vi "COD质控流程 (子VI).vi"(9 "CODMn量程切换":enum32{"H", "L", "AUTO"}(ring)=enum."AUTO", 10 "CODMn":bool) -> (3 "布尔":bool)   [LabVIEW 2016, in "质控单元.lvlib"]
panel:
  out "CODMn中断报警":bool
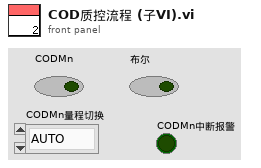
[diagram p1: front panel]
types:
  T1 = enum16{"待机", "启动水样测量", "水样测量中", "启动加标", "启动加标回收", "加标回收测量中", "结束"}
  T2 = cluster{"测量模式":enum16{"水样测量", "标样核查", "零点核查", "跨度核查", "空白测试", "加标回收", "平行样", "校零", "校标"}}
  T3 = enum16{"空闲", "水样测试", "标样核查", "零点核查", "跨度核查", "空白测试", "平行样测试", "质控样", "空白校准", "标样校准", "加标回收"}
  T4 = cluster{"量程":dbl, "检出限":dbl, "加标前水样浓度":dbl, "加标后水样浓度":dbl, "加标水杯定容体积":dbl, "加标母液浓度":dbl, "加标体积":dbl, "加标回收率":dbl}
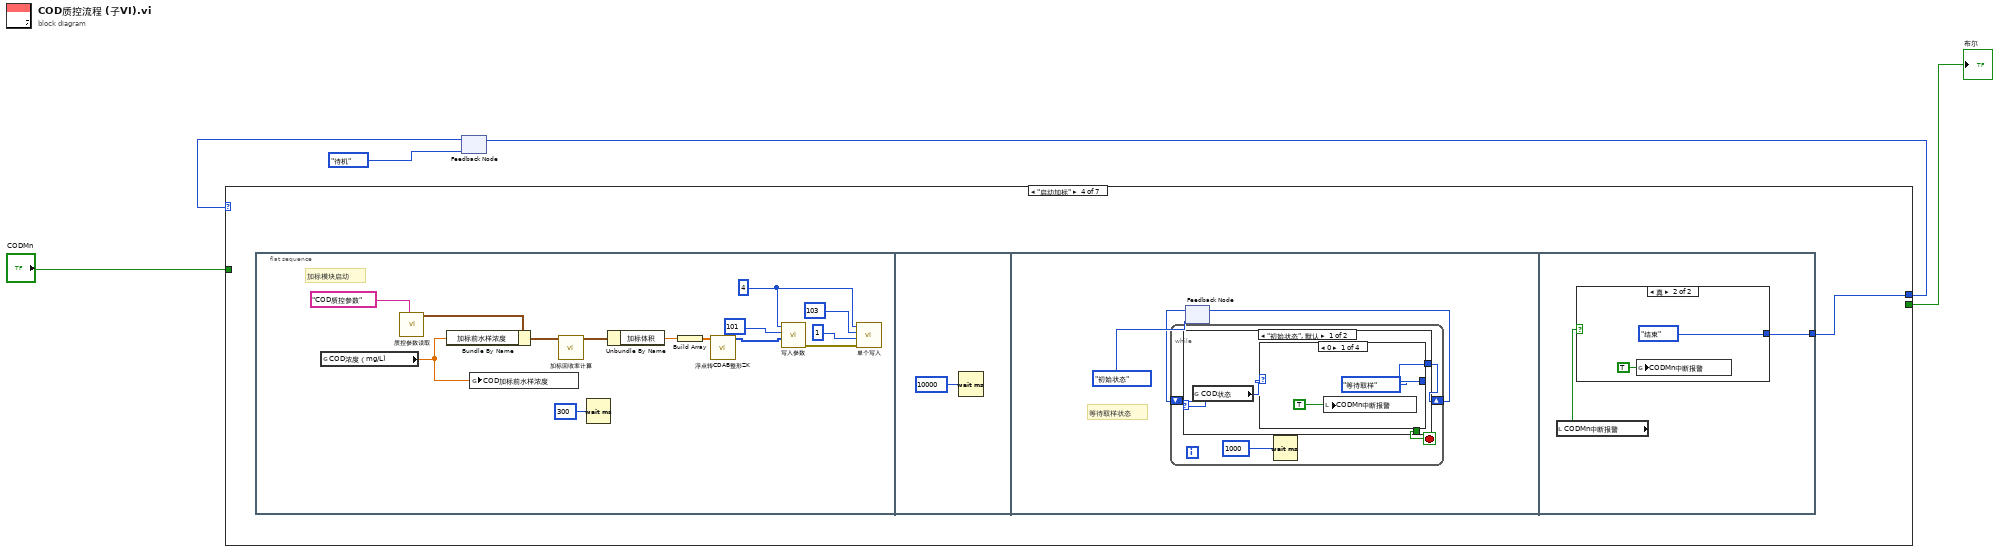
[diagram p0: block diagram]
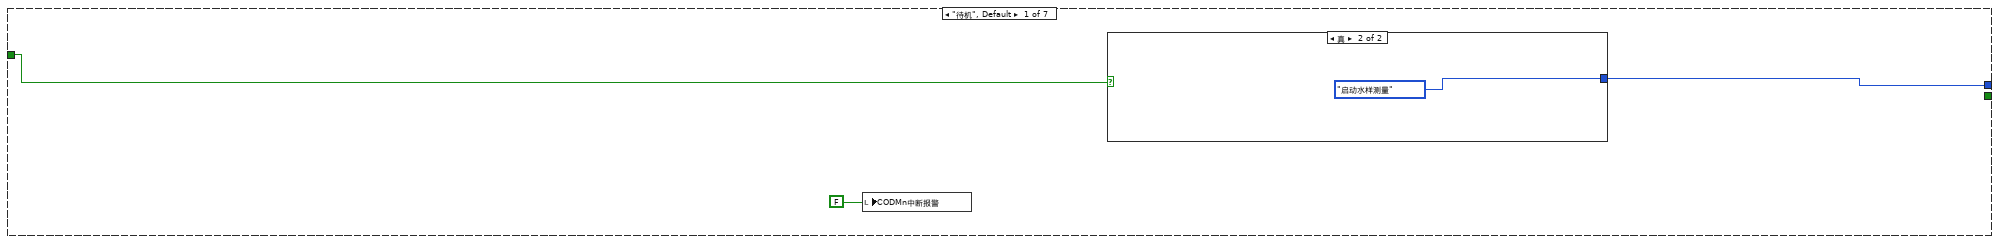
[diagram p2: hidden frame]
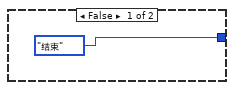
[diagram p3: hidden frame]
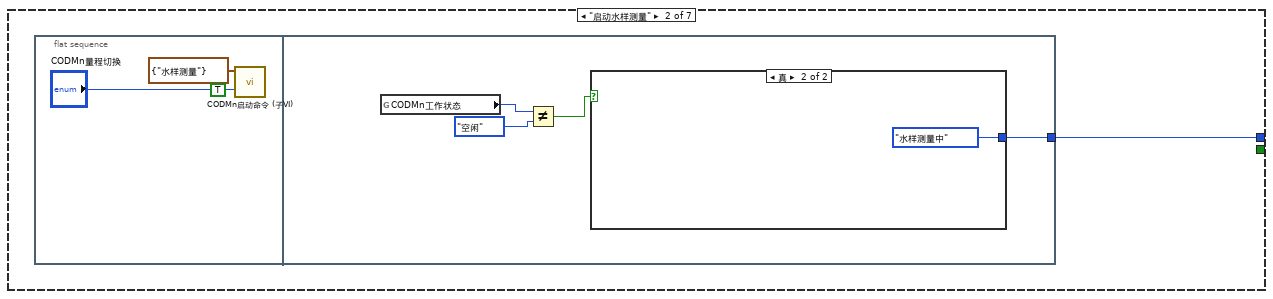
[diagram p4: hidden frame]
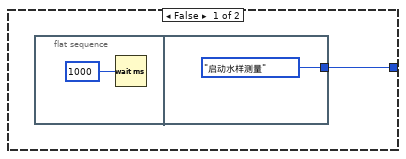
[diagram p5: hidden frame]
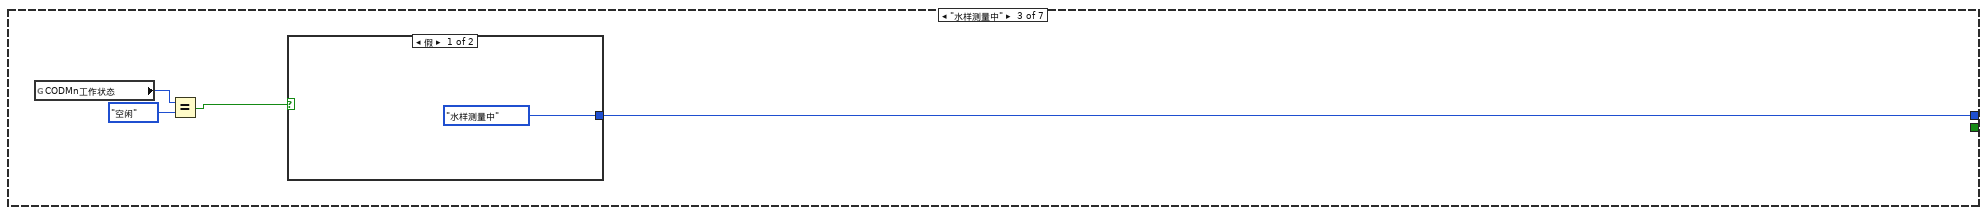
[diagram p6: hidden frame]
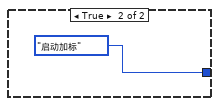
[diagram p7: hidden frame]
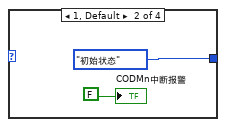
[diagram p8: hidden frame]
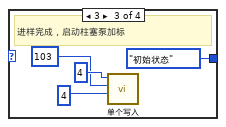
[diagram p9: hidden frame]
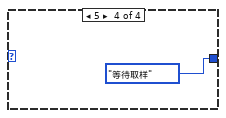
[diagram p10: hidden frame]
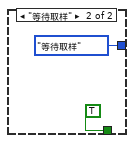
[diagram p11: hidden frame]
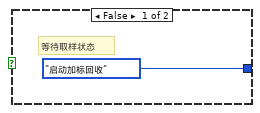
[diagram p12: hidden frame]
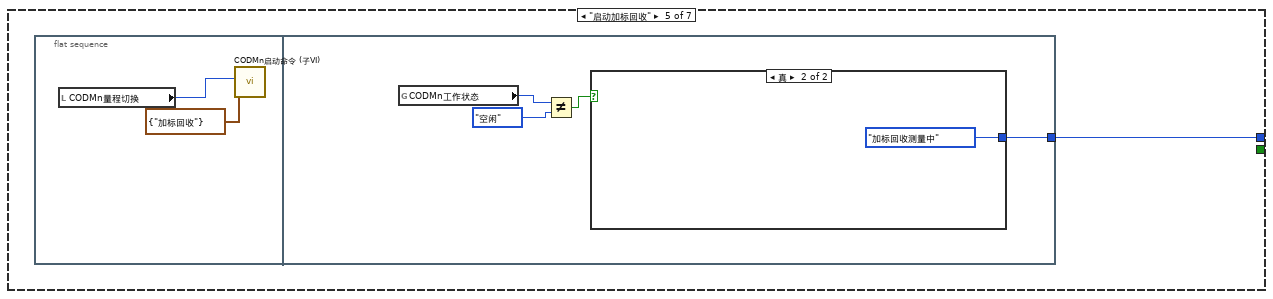
[diagram p13: hidden frame]
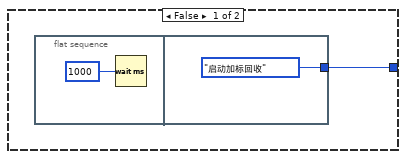
[diagram p14: hidden frame]
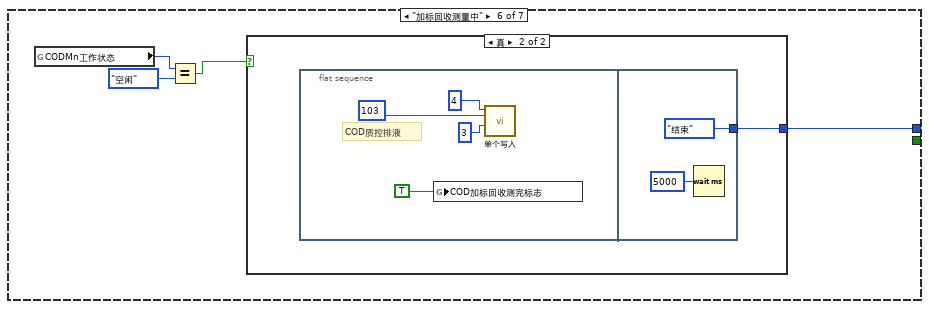
[diagram p15: hidden frame]
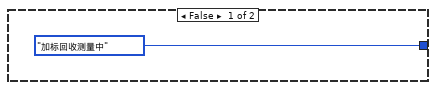
[diagram p16: hidden frame]
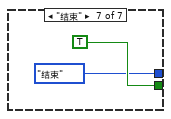
[diagram p17: hidden frame]
diagram:
  n1 = feedback #1(T1."待机") -> (w3:T1)
  n2 = case shown="\"启动加标\"" w3 {
    tunnel: [w8 w11 w26 w29 w70 w84 T1."结束"] -> w4
    tunnel: [_ _ _ _ _ _ TRUE] -> w2
    tunnel: "CODMn" -> [w7 _ _ _ _ _ _]
    frame "待机", Default {
      n3 = local write "CODMn中断报警"(FALSE ("CODMn中断报警")) -> ()
      n4 = case shown="真" w7 {
        tunnel: [T1."结束" T1."启动水样测量"] -> w8
        frame False {
        }
        frame True {
        }
      }
    }
    frame "启动水样测量" {
      n5 = flat-sequence {
        tunnel: [w18] -> w11
        frame #0 {
          n6 = call "CODMn启动命令 (子VI).vi"("强制切换"=TRUE, "CODMn量程切换"="CODMn量程切换", "启动测量模式"=T2 {"测量模式"=enum."水样测量"}) -> ()  [unwired: 8 in, 1 out]
        }
        frame #1 {
          n7 = global read "与CODMn交互全局.vi" "CODMn工作状态"() -> (w17:T3)
          n8 = Not Equal?(x=w17, y=T3."空闲") -> (x != y?=w15:bool)
          n9 = case shown="真" w15 {
            tunnel: [w19 T1."水样测量中"] -> w18
            frame False {
              n10 = flat-sequence {
                tunnel: [T1."启动水样测量"] -> w19
                frame #0 {
                  n11 = Wait (ms)(milliseconds to wait=u32 1000 ("等待时间（毫秒）")) -> ()  [unwired: 1 out]
                }
                frame #1 {
                }
              }
            }
            frame True {
            }
          }
        }
      }
    }
    frame "水样测量中" {
      n12 = global read "与CODMn交互全局.vi" "CODMn工作状态"() -> (w25:T3)
      n13 = Equal?(x=w25, y=T3."空闲") -> (x = y?=w23:bool)
      n14 = case shown="假" w23 {
        tunnel: [T1."水样测量中" T1."启动加标"] -> w26
        frame False {
        }
        frame True {
        }
      }
    }
    frame "启动加标" {
      n15 = flat-sequence {
        tunnel: [w66] -> w29
        frame #0 {
          w31 = u16 4 ("value")
          # "加标模块启动"
          n16 = global read "与CODMn交互全局.vi" "COD浓度（mg/L)"() -> (w32:dbl)
          n17 = call "质控参数读取.vi"("section"="COD质控参数") -> ("参数"=w41:T4)  [unwired: 9 in, 1 out]
          n18 = Bundle By Name(cluster=w41, "加标前水样浓度"=w32) -> (w42:T4)
          n19 = global write "水样浓度全局.vi" "COD加标前水样浓度"(w32) -> ()
          n20 = call "加标回收率计算.vi"("参数"=w42) -> ("参数 out"=w40:T4)  [unwired: 10 in]
          n21 = Wait (ms)(milliseconds to wait=u32 300 ("等待时间（毫秒）")) -> ()  [unwired: 1 out]
          n22 = Unbundle By Name(w40) -> ("加标体积"=w33:dbl)
          n23 = Build Array(w33) -> (w39:dbl[])
          n24 = call "浮点转CDAB整形ZK.vi"("浮点数"=w39) -> ("CDAB整形输出"=w34:u16[])  [unwired: 10 in]
          n25 = call "写入参数.vi"("values"=w34, "starting address"=u16 101, "Slave ID"=w31) -> ("error out"=w38:errorcluster)  [unwired: 8 in]
          n26 = call "单个写入.vi"("Error in"=w38, "value"=u16 1, "address"=u16 103, "Slave ID"=w31) -> ()  [unwired: 7 in, 1 out]
        }
        frame #1 {
          n27 = Wait (ms)(milliseconds to wait=u32 10000 ("等待时间（毫秒）")) -> ()  [unwired: 1 out]
        }
        frame #2 {
          # "等待取样状态"
          n28 = feedback #2(enum16{"初始状态", "等待取样"}."初始状态") -> (w46:enum16{"初始状态", "等待取样"})
          n29 = while {
            shift-right: [w50] -> w45
            shift-left: w46 -> [w51]
            stop <- w49 stop-if-true
            n30 = case shown="\"初始状态\", 默认" w51 {
              tunnel: [w53 enum16{"初始状态", "等待取样"}."等待取样"] -> w50
              tunnel: [_ TRUE] -> w49
              frame "初始状态", Default {
                n31 = global read "加标回收状态全局变量.vi" "COD状态"() -> (w52:u16)
                n32 = case shown="0" w52 {
                  tunnel: [enum16{"初始状态", "等待取样"}."等待取样" enum16{"初始状态", "等待取样"}."初始状态" enum16{"初始状态", "等待取样"}."初始状态" enum16{"初始状态", "等待取样"}."等待取样"] -> w53
                  frame 0 {
                    n33 = local write "CODMn中断报警"(TRUE ("氨氮中断报警")) -> ()
                  }
                  frame 1, Default {
                    "CODMn中断报警" <- FALSE ("总氮中断报警")
                  }
                  frame 3 {
                    # "进样完成，启动柱塞泵加标"
                    n34 = call "单个写入.vi"("value"=u16 4, "address"=u16 103, "Slave ID"=u8 4) -> ()  [unwired: 8 in, 1 out]
                  }
                  frame 5 {
                  }
                }
              }
              frame "等待取样" {
              }
            }
            n35 = Wait (ms)(milliseconds to wait=u32 1000 ("等待时间（毫秒）")) -> ()  [unwired: 1 out]
          }
          n36 = feedback-in #2(w45) -> ()
        }
        frame #3 {
          n37 = local read "CODMn中断报警"() -> (w65:bool)
          n38 = case shown="真" w65 {
            tunnel: [T1."启动加标回收" T1."结束"] -> w66
            frame False {
              # "等待取样状态"
            }
            frame True {
              n39 = global write "质控中断报警全局.vi" "CODMn中断报警"(TRUE ("CODMn中断报警")) -> ()
            }
          }
        }
      }
    }
    frame "启动加标回收" {
      n40 = flat-sequence {
        tunnel: [w76] -> w70
        frame #0 {
          n41 = local read "CODMn量程切换"() -> (w72:enum32{"H", "L", "AUTO"})
          n42 = call "CODMn启动命令 (子VI).vi"("CODMn量程切换"=w72, "启动测量模式"=T2 {"测量模式"=enum."加标回收"}) -> ()  [unwired: 9 in, 1 out]
        }
        frame #1 {
          n43 = global read "与CODMn交互全局.vi" "CODMn工作状态"() -> (w75:T3)
          n44 = Not Equal?(x=w75, y=T3."空闲") -> (x != y?=w73:bool)
          n45 = case shown="真" w73 {
            tunnel: [w77 T1."加标回收测量中"] -> w76
            frame False {
              n46 = flat-sequence {
                tunnel: [T1."启动加标回收"] -> w77
                frame #0 {
                  n47 = Wait (ms)(milliseconds to wait=u32 1000 ("等待时间（毫秒）")) -> ()  [unwired: 1 out]
                }
                frame #1 {
                }
              }
            }
            frame True {
            }
          }
        }
      }
    }
    frame "加标回收测量中" {
      n48 = global read "与CODMn交互全局.vi" "CODMn工作状态"() -> (w83:T3)
      n49 = Equal?(x=w83, y=T3."空闲") -> (x = y?=w81:bool)
      n50 = case shown="真" w81 {
        tunnel: [T1."加标回收测量中" w86] -> w84
        frame False {
        }
        frame True {
          n51 = flat-sequence {
            tunnel: [T1."结束"] -> w86
            frame #0 {
              # "COD质控排液"
              n52 = global write "质控测完标志全局 1.vi" "COD加标回收测完标志"(TRUE ("COD加标回收测完标志")) -> ()
              n53 = call "单个写入.vi"("value"=u16 3, "address"=u16 103, "Slave ID"=u8 4) -> ()  [unwired: 8 in, 1 out]
            }
            frame #1 {
              n54 = Wait (ms)(milliseconds to wait=u32 5000 ("等待时间（毫秒）")) -> ()  [unwired: 1 out]
            }
          }
        }
      }
    }
    frame "结束" {
    }
  }
  "布尔" <- w2
  n55 = feedback-in #1(w4) -> ()
